vi "Build Datagram.vi"(4 "destination address":u32, 5 "transfer id":i32, 6 "destination port":u16, 7 "transfer group id":i32, 8 "error in (no error)":errorcluster, 10 "transfer data":string, 11 "UDPlog Transceiver in":refnum<class "UDPlog Transceiver.lvclass">) -> (0 "error out":errorcluster, 2 "datagram":string, 3 "UDPlog Transceiver out":refnum<class "UDPlog Transceiver.lvclass">)   [LabVIEW 2023, in "UDPlog.lvlib" / "UDPlog Transceiver.lvclass"]
uses:
  UDPlog Transceiver.lvclass
  UDPlog Transceiver.lvclass/UDPlog Transceiver.ctl
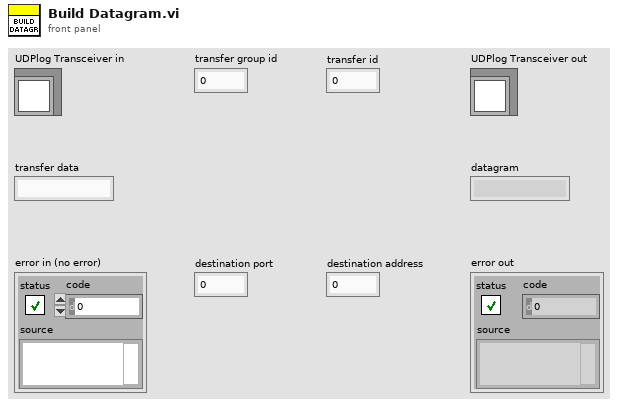
[diagram p1: front panel]
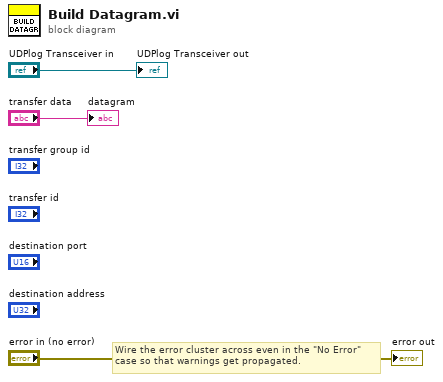
[diagram p0: block diagram]
diagram:
  # "Wire the error cluster across even in the \"No Error\"\ncase so that warnings get propagated."
  "error out" <- "error in (no error)"
  "UDPlog Transceiver out" <- "UDPlog Transceiver in"
  "datagram" <- "transfer data"
